vi "Default Instrument Setup.vi"(8 "error in (no error)":errorcluster, 11 "VISA resource name":refnum<visa-resource-name>) -> (0 "error out":errorcluster, 3 "VISA resource name out":refnum<visa-resource-name>)   [LabVIEW 2017, in "GP22_TDC_Arduinoed.lvlib"]
doc: "Set up the TDC with default settings. \n\nOptions:\nDouble resolution - doubles the resolution of the TDC but causes the device to miss stop events faster than around 30ns. \nAuto calibrate - Allow the TDC to take care of its own calibration and return calculated results. This takes far longer than measuring raw data and post processing it."
uses:
  GP22_TDC_Arduinoed.lvlib
  Public/Globals.vi
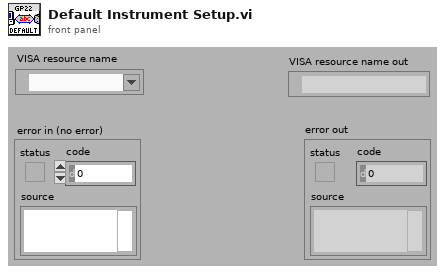
[diagram p1: front panel]
types:
  T1 = typedef "GP22_TDC_Arduinoed.lvlib/Registers.ctl" = cluster{"Reg0":u32, "Reg1":u32, "Reg2":u32, "Reg3":u32, "Reg4":u32, "Reg5":u32, "Reg6":u32}
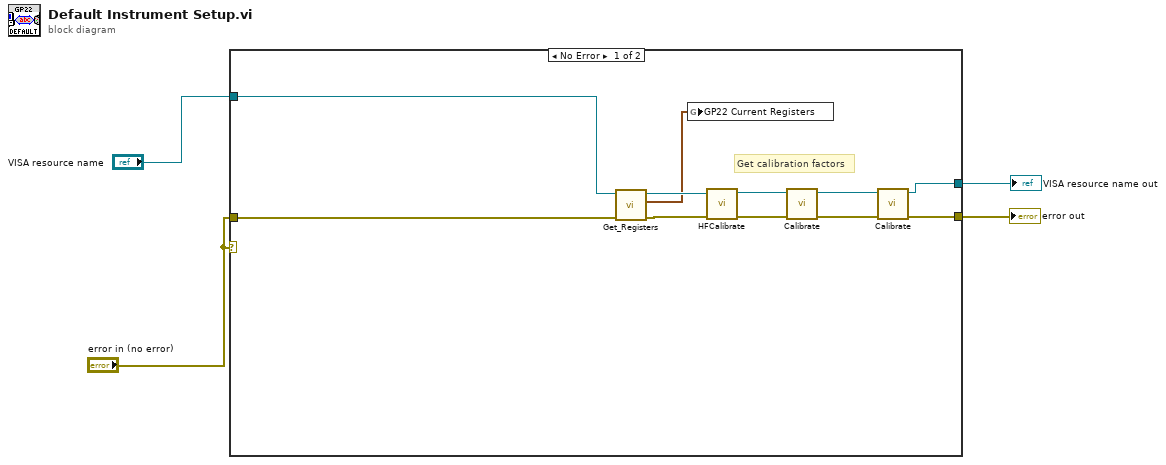
[diagram p0: block diagram]
diagram:
  n1 = case shown="No Error" "error in (no error)" {
    tunnel: "error in (no error)" -> [w6 w17]
    tunnel: [w13 w17] -> w4
    tunnel: [w10 w16] -> w2
    tunnel: "VISA resource name" -> [w9 w16]
    frame No Error {
      # "Get calibration factors"
      n2 = call "Get_Registers.vi"("error in (no error)"=w6, "VISA in"=w9) -> ("error out"=w7:errorcluster, "Registers"=w5:T1, "VISA out"=w8:refnum<visa-resource-name>)  [unwired: 3 in]
      n3 = global write "Globals.vi" "GP22 Current Registers"(w5) -> ()
      n4 = call "HFCalibrate.vi"("error in (no error)"=w7, "VISA resource name"=w8) -> ("error out"=w12:errorcluster, "VISA resource name out"=w11:refnum<visa-resource-name>)  [unwired: 5 in, 2 out]
      n5 = call "Calibrate.vi"("error in (no error)"=w12, "VISA resource name"=w11) -> ("error out"=w14:errorcluster, "VISA resource name out"=w15:refnum<visa-resource-name>)  [unwired: 5 in, 2 out]
      n6 = call "Calibrate.vi"("error in (no error)"=w14, "VISA resource name"=w15) -> ("error out"=w13:errorcluster, "VISA resource name out"=w10:refnum<visa-resource-name>)  [unwired: 5 in, 2 out]
    }
    frame Error {
    }
  }
  "error out" <- w4
  "VISA resource name out" <- w2
